vi "New.vi"(8 "Error in (no error)":errorcluster, 11 "Reference in":refnum<class "Static TestSuite.lvclass">) -> (0 "Error out":errorcluster, 3 "Reference out":refnum<class "Static TestSuite.lvclass">)   [LabVIEW 2013, in "Static TestSuite.lvclass"]
uses:
  Static TestSuite.lvclass
  LocationOutsideClassRoot/LocationOutsideClassRoot.lvclass
  Classes/TestSuite/TestSuite.lvclass
  Classes/TestCase/TestCase.lvclass
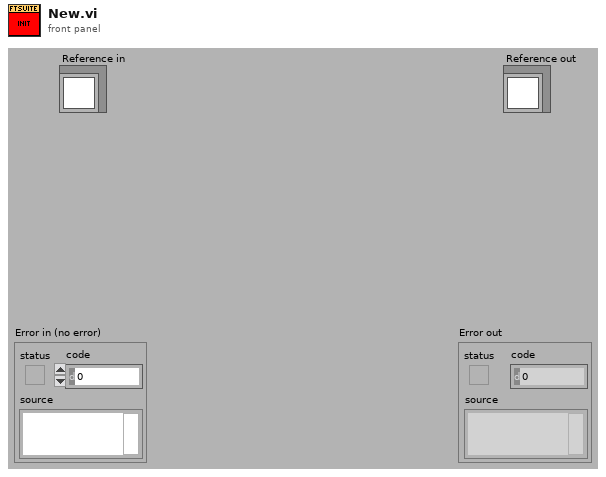
[diagram p1: front panel]
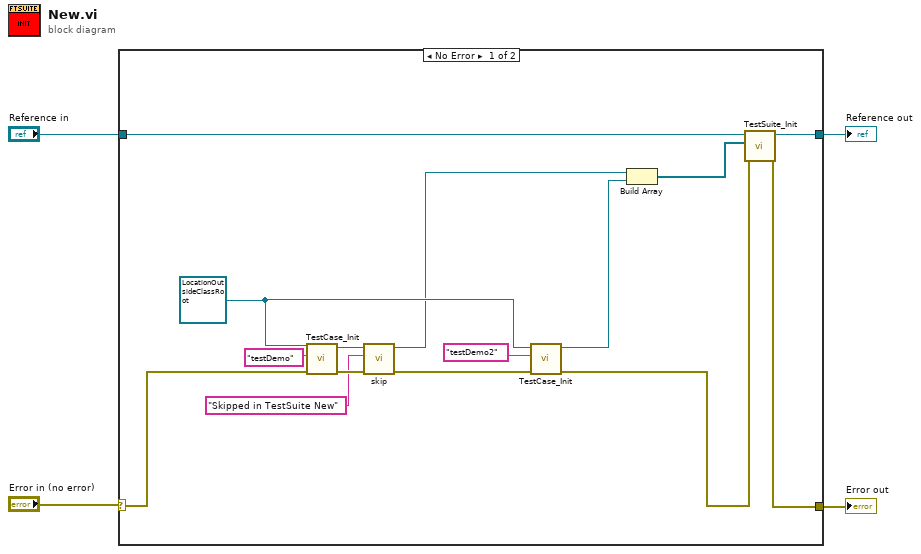
[diagram p0: block diagram]
diagram:
  n1 = case shown="No Error" "Error in (no error)" {
    selector: "Error in (no error)" -> [w17 w20]
    tunnel: [w16 w21] -> w4
    tunnel: "Reference in" -> [w18 w21]
    tunnel: [w19 w20] -> w1
    frame No Error {
      w13 = refnum<class "LocationOutsideClassRoot.lvclass"> refnum ("LocationOutsideClassRoot.lvclass")
      n2 = call "TestCase_Init.vi"("error in (no error)"=w17, "methodName (\"runTest\")"="testDemo", "TestCase in"=w13) -> ("error out"=w9:errorcluster, "TestCase out"=w7:refnum<class "LocationOutsideClassRoot.lvclass">)  [unwired: 7 in]
      n3 = call "skip.vi"("error in (no error)"=w9, "skipMessage"="Skipped in TestSuite New", "TestCase in"=w7) -> ("error out"=w8:errorcluster, "TestCase out"=w6:refnum<class "LocationOutsideClassRoot.lvclass">)  [unwired: 7 in]
      n4 = call "TestCase_Init.vi"("error in (no error)"=w8, "methodName (\"runTest\")"="testDemo2", "TestCase in"=w13) -> ("error out"=w11:errorcluster, "TestCase out"=w10:refnum<class "LocationOutsideClassRoot.lvclass">)  [unwired: 7 in]
      n5 = Build Array(w6, w10) -> (w15:refnum<class "LocationOutsideClassRoot.lvclass">[])
      n6 = call "TestSuite_Init.vi"("error in (no error)"=w11, "tests (none)"=w15, "TestSuite in"=w18) -> ("error out"=w19:errorcluster, "TestSuite out"=w16:refnum<class "Static TestSuite.lvclass">)  [unwired: 7 in]
    }
    frame Error {
    }
  }
  "Reference out" <- w4
  "Error out" <- w1
